vi "SEA_9811_RT_FIFO_processor.vi"(8 "error in (no error)":errorcluster, 9 "Number of Elements":u32, 10 "9811 Data in":u64[](array[numeric]), 11 "SEA9811_RT_data in":T1 {"Tx"."Tx Refs (Data,Trig)"."Data Reference" format="%.0x"}) -> (0 "error out":errorcluster, 3 "SEA9811_RT_data out":T1 {"Tx"."Tx Refs (Data,Trig)"."Data Reference" format="%.0x"})   [LabVIEW 2015]
doc: "processes elements from FPGA and puts ARINC word and timestamp into DBL array"
uses:
  Typdefs/SEA9811_RT_data_cluster.ctl
  <userlib>/_FPGA Interface Advanced Tools/FPGA Interface Base/FPGA Interface Base.lvclass
  Typdefs/FPGA ref.ctl
  Typdefs/channel.ctl
  Typdefs/received word.ctl
  Typdefs/SEA9811_FPGA_FP_Addresses.ctl
  <vilib>/NI Veristand/Custom Device API/Block Data Reference.ctl
  <vilib>/NI Veristand/Custom Device API/Data Reference.ctl
  <userlib>/FPGA Timekeeper 1.1b0/FPGA Timekeeper.lvlib
  <vilib>/NI VeriStand/Custom Device API/Custom Device API.lvlib
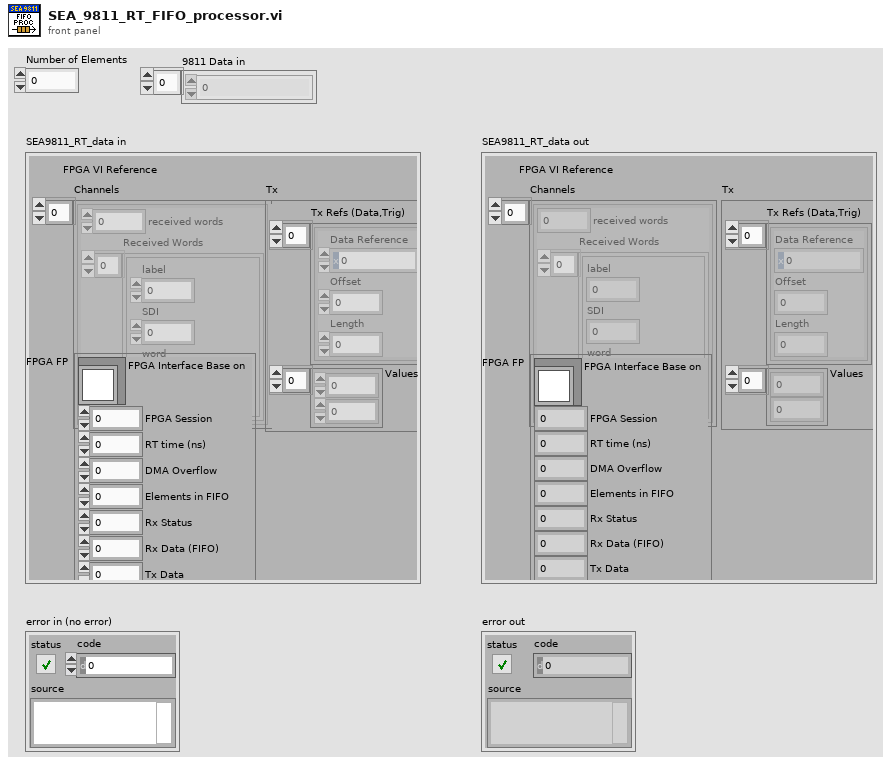
[diagram p1: front panel]
types:
  T1 = typedef "SEA9811_RT_data_cluster.ctl" = cluster{"FPGA VI Reference":T2, "Channels":T3[], "FPGA FP":T5, "Tx":cluster{"Tx Refs (Data,Trig)":T6[], "Values":dbl[]}}
  T2 = typedef "FPGA ref.ctl" = refnum<k20>
  T3 = typedef "channel.ctl" = cluster{"received words":u32, "Received Words":T4[]}
  T4 = typedef "received word.ctl" = cluster{"label":u8, "SDI":u8, "word":u32, "timestamp":dbl}
  T5 = typedef "SEA9811_FPGA_FP_Addresses.ctl" = cluster{"FPGA Interface Base on":refnum<class "FPGA Interface Base.lvclass">, "FPGA Session":u32, "RT time (ns)":u32, "DMA Overflow":u32, "Elements in FIFO":u32, "Rx Status":u32, "Rx Data (FIFO)":u32, "Tx Data":u32, "Transmit Data":u32}
  T6 = typedef "Custom Device API.lvlib/Block Data Reference.ctl" = cluster{"Data Reference":T7, "Offset":u64, "Length":u64}
  T7 = typedef "Custom Device API.lvlib/Data Reference.ctl" = i32
  T8 = typedef "ARINC word cluster.ctl" = cluster{"ARINC word":T9, "Label":u8, "SDI":u8, "Data":u32, "Parity":bool, "timestamp (DBL)":dbl}
  T9 = typedef "ARINC word.ctl" = u32
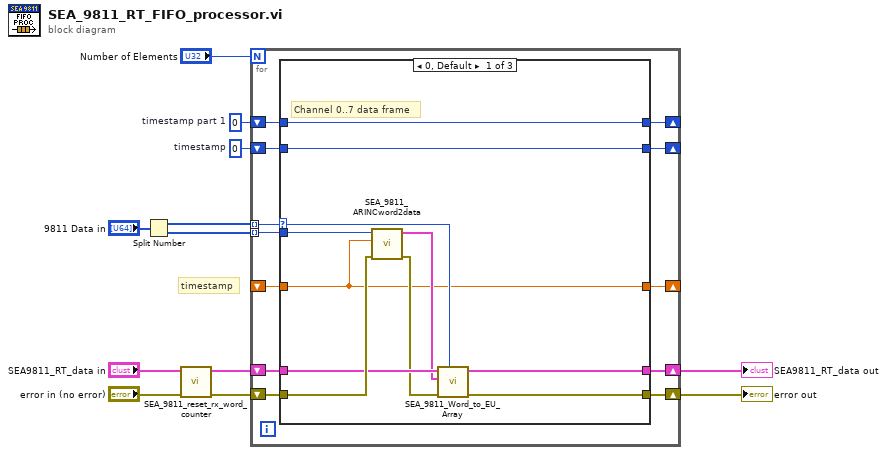
[diagram p0: block diagram]
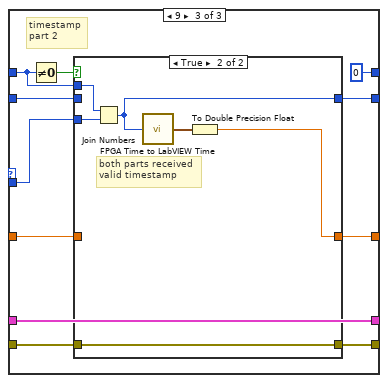
[diagram p3: hidden frame]
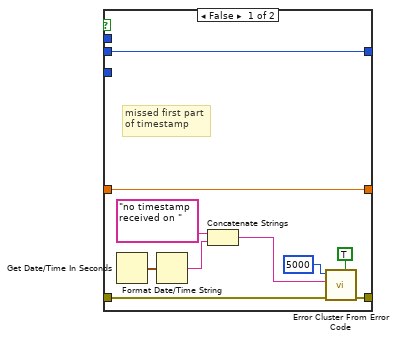
[diagram p4: hidden frame]
diagram:
  w8 = u32 0  # timestamp part 1
  w10 = u32 0  # timestamp
  # "timestamp"
  n1 = Split Number(x="9811 Data in") -> (hi(x)=w12:u32[], lo(x)=w11:u32[])
  n2 = call "SEA_9811_reset_rx_word_counter.vi"("error in (no error)"="error in (no error)", "SEA9811_RT_data in"="SEA9811_RT_data in") -> ("error out"=w2:errorcluster, "SEA9811_RT_data out"=w4:T1)  [unwired: 8 in]
  n3 = for {
    N: "Number of Elements" -> [_]
    tunnel: w12 -> [w24] mode=indexing
    tunnel: w11 -> [w21] mode=indexing
    shift-right: [w23] -> _
    shift-left: w10 -> [w22]
    shift-right: [w20] -> _
    shift-left: w8 -> [w19]
    shift-right: [w17] -> w7
    shift-left: w2 -> [w18]
    shift-right: [w16] -> _
    shift-left: _ -> [w15]
    shift-right: [w13] -> w6
    shift-left: w4 -> [w14]
    n4 = case shown="0, Default" w24 {
      selector: w24 -> [w31 _ _]
      tunnel: [w35 w39 w46] -> w23
      tunnel: w22 -> [w35 w39 w47]
      tunnel: w21 -> [w26 w40 w48]
      tunnel: [w34 w40 u32 0] -> w20
      tunnel: w19 -> [w34 _ w49]
      tunnel: w18 -> [w33 w37 w45]
      tunnel: [w28 w37 w44] -> w17
      tunnel: [w25 w38 w43] -> w16
      tunnel: w15 -> [w25 w38 w42]
      tunnel: w14 -> [w32 w36 w41]
      tunnel: [w27 w36 w41] -> w13
      frame 0, Default {
        # "Channel 0..7 data frame"
        n5 = call "SEA_9811_ARINCword2data.vi"("error in (no error)"=w33, "timestamp (DBL) in"=w25, "ARINC word in"=w26) -> ("error out"=w29:errorcluster, "ARINC word out"=w30:T8)  [unwired: 7 in]
        n6 = call "SEA_9811_Word_to_EU_Array.vi"("Channel"=w31, "error in (no error)"=w29, "ARINC word in"=w30, "SEA9811_RT_data in"=w32) -> ("error out"=w28:errorcluster, "SEA9811_RT_data out"=w27:T1)  [unwired: 6 in]
      }
      frame 8 {
        # "timestamp\npart 1"
      }
      frame 9 {
        # "timestamp\npart 2"
        n7 = Not Equal To 0?(x=w49) -> (x != 0?=w50:bool)
        n8 = case shown="True" w50 {
          tunnel: w49 -> [_ w67]
          tunnel: w48 -> [_ w66]
          tunnel: w47 -> [w61 _]
          tunnel: [w61 w64] -> w46
          tunnel: w45 -> [w58 w65]
          tunnel: [w57 w65] -> w44
          tunnel: [w52 w62] -> w43
          tunnel: w42 -> [w52 _]
          frame False {
            # "missed first part\nof timestamp"
            n9 = Get Date/Time In Seconds() -> (seconds since 1Jan1904=w56:timestamp)
            n10 = Format Date/Time String(seconds (now)=w56) -> (date/time string=w54:string)  [unwired: 2 in]
            n11 = Concatenate Strings("no timestamp received on " ("string"), w54) -> (w53:string)
            n12 = call <vilib>:"Error Cluster From Error Code.vi"("is warning? (False)"=TRUE, "error in (no error)"=w58, "error message (\"\")"=w53, "error code (0)"=5000) -> ("error out"=w57:errorcluster)  [unwired: 5 in]
          }
          frame True {
            # "both parts received\nvalid timestamp"
            n13 = Join Numbers(hi=w67, lo=w66) -> ((hi.lo)=w64:u64)
            n14 = call <userlib>:"FPGA Time to LabVIEW Time.vi"("FPGA time (ns)"=w64) -> ("LabVIEW time"=w63:timestamp)
            n15 = To Double Precision Float(number=w63) -> (double precision float=w62:dbl)
          }
        }
      }
    }
  }
  "SEA9811_RT_data out" <- w6
  "error out" <- w7
